vi "Set VI Ref.vi"(8 "error in":errorcluster, 11 "vi ref":refnum<vi>) -> (0 "error out":errorcluster, 3 "vi id":string)   [LabVIEW 2026, in "G-AI Core.lvlib"]
doc: "Stores a VI reference for later use and returns a string with a unique vi id to return to the LLM for later use."
uses:
  G-AI Core.lvlib
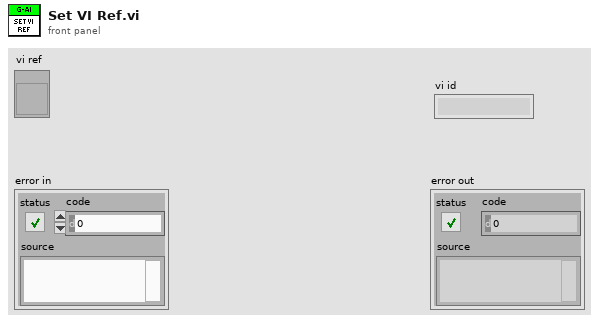
[diagram p1: front panel]
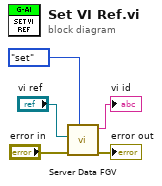
[diagram p0: block diagram]
diagram:
  n1 = call "Server Data FGV.vi"("mode"=enum16{"get", "set", "reset"}."set", "error in"="error in", "data in"="vi ref") -> ("error out"=→"error out":errorcluster, "name out"=→"vi id":string)  [unwired: 5 in, 2 out]
